vi "play_wav.vi"(8 "error in":errorcluster, 11 "problem":enum16{"OK", "Warning", "Error"}(ring)=enum."Error") -> (0 "error out":errorcluster, 3 "status":bool, 4 "path":path)   [LabVIEW 2019]
panel:
  # "Sub-VI to play a WAV file."
  # "The default audio device must be available before this sub VI is called."
  # "Otherwise \"Play Sound File VI\" returns error code 8400 even after the device is made available."
  # "In such case this sub VI and all other VIs that calls this sub VI must be close!"
  # "\"Play Sound File VI\" gets stuck if the sound is played successfully once and then the device becomes unavailable."
  # "In such case the device must be made available to let \"Play Sound File VI\" finish (or kill LabVIEW)!"
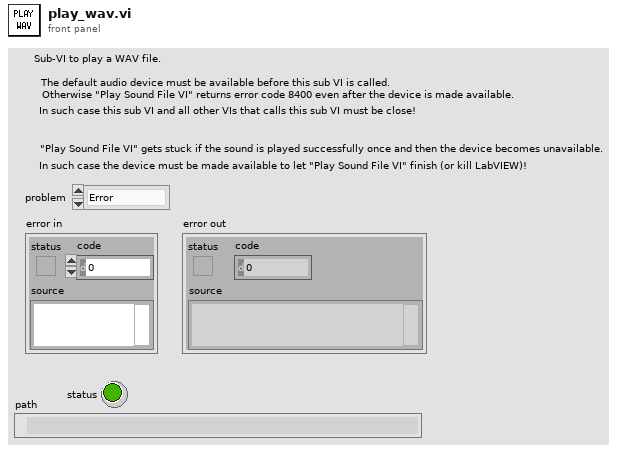
[diagram p1: front panel]
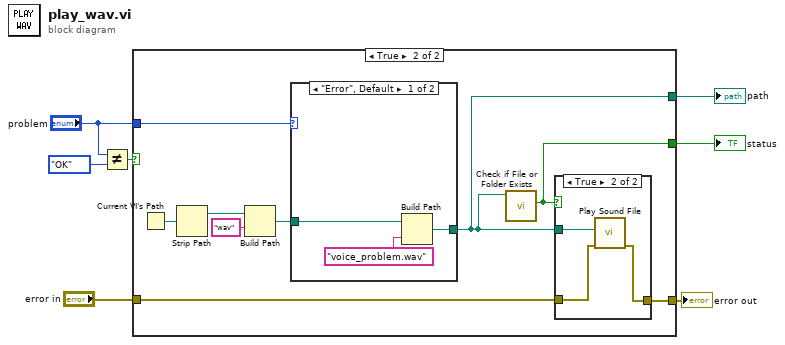
[diagram p0: block diagram]
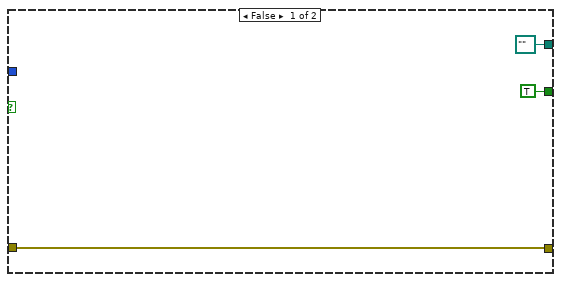
[diagram p2: hidden frame]
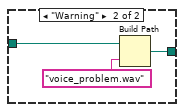
[diagram p4: hidden frame]
diagram:
  n1 = Not Equal?(x="problem", y=enum16{"OK", "Warning", "Error"}."OK") -> (x != y?=w6:bool)
  n2 = case shown="True" w6 {
    tunnel: "problem" -> [_ w19]
    tunnel: "error in" -> [w10 w14]
    tunnel: [w10 w13] -> w3
    tunnel: [TRUE ("file or folder exists?") w12] -> w2
    tunnel: [path "" ("appended path") w11] -> w1
    frame False {
    }
    frame True {
      n3 = Current VI's Path() -> (path=w18:path)
      n4 = Strip Path(path=w18) -> (stripped path=w17:path)  [unwired: 1 out]
      n5 = Build Path(base path=w17, name or relative path="wav") -> (appended path=w15:path)
      n6 = case shown="\"Error\", Default" w19 {
        tunnel: [w24 w28] -> w11
        tunnel: w15 -> [w26 w27]
        frame "Error", Default {
          n7 = Build Path(base path=w26, name or relative path="voice_problem.wav") -> (appended path=w24:path)
        }
        frame "Warning" {
          n8 = Build Path(base path=w27, name or relative path="voice_problem.wav") -> (appended path=w28:path)
        }
      }
      n9 = call <vilib>:"Check if File or Folder Exists.vi"("path"=w11) -> ("file or folder exists?"=w12:bool)  [unwired: 8 in, 2 out]
      n10 = case shown="True" w12 {
        tunnel: w14 -> [w20 w23]
        tunnel: [w20 w22] -> w13
        tunnel: w11 -> [_ w21]
        frame False {
        }
        frame True {
          n11 = call <vilib>:"Play Sound File.vi"("error in (no error)"=w23, "path"=w21) -> ("error out"=w22:errorcluster)  [unwired: 8 in, 1 out]
        }
      }
    }
  }
  "error out" <- w3
  "status" <- w2
  "path" <- w1
